vi "Test Animal Can Sleep after Eating.vi"(8 "error in (no error)":errorcluster, 11 "Animal Test In":refnum<class "Animal Test.lvclass">) -> (0 "error out":errorcluster, 3 "Animal Test Out":refnum<class "Animal Test.lvclass">)   [LabVIEW 2020, in "Animal Test.lvclass"]
doc: "Test Animal can sleep after eating"
uses:
  Animal Test.lvclass
  C:/Program Files (x86)/National Instruments/LabVIEW 2020/vi.lib/Astemes/LUnit/Test Case.lvclass
  Animal Test.lvclass/Animal Test.ctl
  <vilib>/Astemes/LUnit/Test Case.lvclass/Test Case.ctl
  8d3ae716-8c5c-4c5b-bc24-4668972be4de.vi
  <vilib>/Astemes/LUnit/Append Pass Result.vi
  <vilib>/Astemes/LUnit/Append Fail Result.vi
  <vilib>/Astemes/LUnit/Describe Comparison.vi
  <vilib>/Astemes/LUnit/Compare Variants.vi
  <vilib>/Astemes/LUnit/Run In UI.vi
  <vilib>/Utility/error.llb/Clear Errors.vi
  <vilib>/Astemes/LUnit/Describe Variant.vi
  Animal Classes/Animal/Animal.lvclass
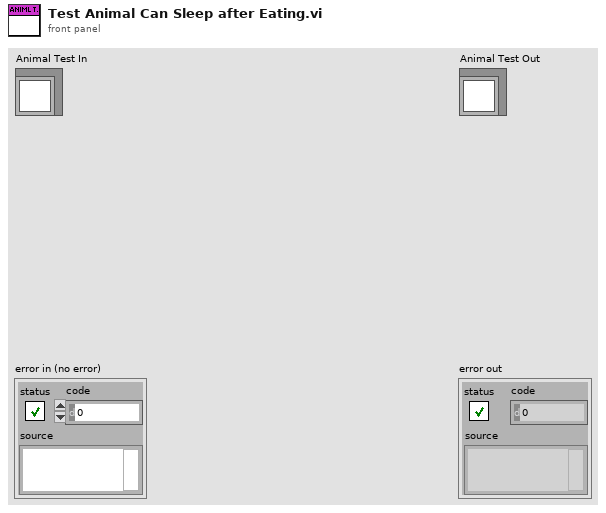
[diagram p1: front panel]
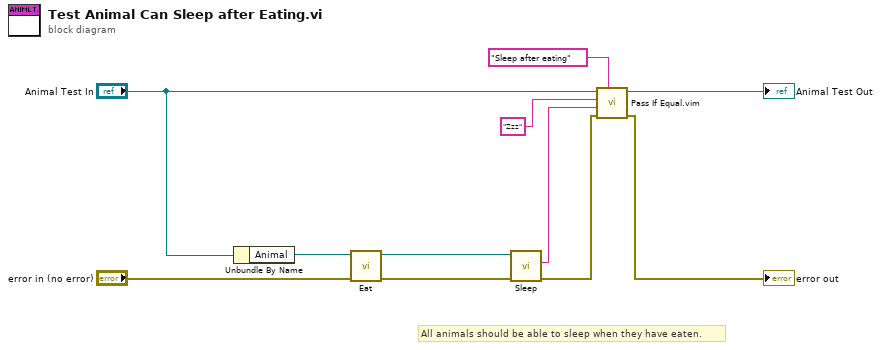
[diagram p0: block diagram]
diagram:
  # "All animals should be able to sleep when they have eaten."
  n1 = Unbundle By Name("Animal Test In") -> ("Animal"=w11:refnum<class "Animal.lvclass">)
  n2 = call-dynamic "Eat.vi"("error in (no error)"="error in (no error)", "Animal In"=w11) -> ("error out"=w2:errorcluster, "Animal Out"=w10:refnum<class "Animal.lvclass">)  [unwired: 7 in, 1 out]
  n3 = call-dynamic "Sleep.vi"("error in (no error)"=w2, "Animal in"=w10) -> ("error out"=w7:errorcluster, "Result"=w4:string)  [unwired: 7 in, 1 out]
  n4 = call "Pass If Equal.vim"("Description"="Sleep after eating", "error in (no error)"=w7, "Actual"=w4, "Expected"="Zzz" ("Result"), "LUnit Test Case In"="Animal Test In") -> ("error out"=→"error out":errorcluster, "LUnit Test Case Out"=→"Animal Test Out":refnum<class "Animal Test.lvclass">)  [unwired: 5 in]
